vi "soundwave_generator_v01_only_player.vi"() -> ()   [LabVIEW 2019]
uses:
  <vilib>/sound2/lvsound2.llb/Sound Data Format.ctl
  <vilib>/sound2/lvsound2.llb/Sampling Mode.ctl
  <vilib>/Platform/TimedLoop/XDataNode/timing_clust.ctl
  <vilib>/Platform/TimedLoop/XDataNode/nitl_modes.ctl
  <vilib>/Platform/TimedLoop/XDataNode/wakeup.ctl
  <vilib>/sound2/lvsound2.llb/Sound Output Set Volume (Single).vi
  <vilib>/sound2/lvsound2.llb/Sound Output Write (DBL Single).vi
  <vilib>/platform/TimedLoop/XDataNode/XDataNode.xnode
  <vilib>/Platform/TimedLoop/XDataNode/XDNodeRunTimeDep.lvlib
panel:
  in  "frequency 2":dbl=440.0
  in  "volume 2":dbl(slide)=50.0 scale=0.0..100.0
  in  "play button 2":bool
  in  "play button 1":bool
  in  "frequency 1":dbl=440.0
  in  "volume 1":dbl(slide)=50.0 scale=0.0..100.0
  in  "stop":bool
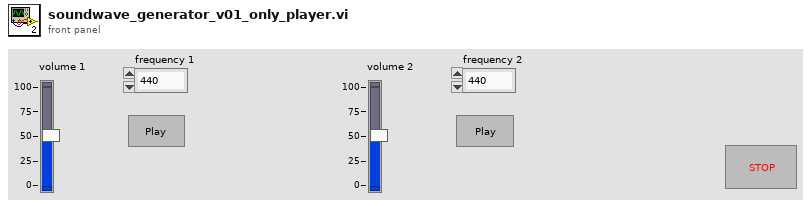
[diagram p1: front panel]
types:
  T1 = typedef "Sound Data Format.ctl" = cluster{"sample rate (S/s)":dbl, "number of channels":i32, "bits per sample":i32}
  T2 = typedef "XDNodeRunTimeDep.lvlib/timing_clust.ctl" = cluster{"Expected End [f-1]":u64, "Actual End [f-1]":u64, "Finished Late? [f-1]":bool, "Expected End [i-1]":u64, "Actual End [i-1]":u64, "Finished Late? [i-1]":bool, "Expected Start [i]":u64, "Actual Start [i]":u64, "Expected Start [f]":u64, "Actual Start [f]":u64, "Source Name":string, "Structure Name":string, "Period":i64, "Deadline":i64, "Offset":i64, "Start":i64, "Priority":i32, "Timeout":i32, "Mode":T3, "Wakeup Reason":T4, "Error":errorcluster, "Source Type":string, "Secondary Source Type":string, "Global End Time":u64, "Global Start Time":u64, "Frame Duration":u64, "Iteration Duration":u64, "Assigned CPU":i32, "I/O Scan Engine Mode":u32}
  T3 = typedef "XDNodeRunTimeDep.lvlib/nitl_modes.ctl" = enum32{"No Change", "Process missed periods, maintain original phase", "Discard missed periods, maintain original phase", "Process missed periods, ignore original phase", "Discard missed periods, ignore original phase"}
  T4 = typedef "XDNodeRunTimeDep.lvlib/wakeup.ctl" = enum32{"Normal", "Aborted", "Asynchronous wakeup", "Timing source error", "Timed loop error", "Timeout"}
  T5 = typedef "Sampling Mode.ctl" = i32
  T6 = typedef "Sound Output Task ID.ctl" = u32
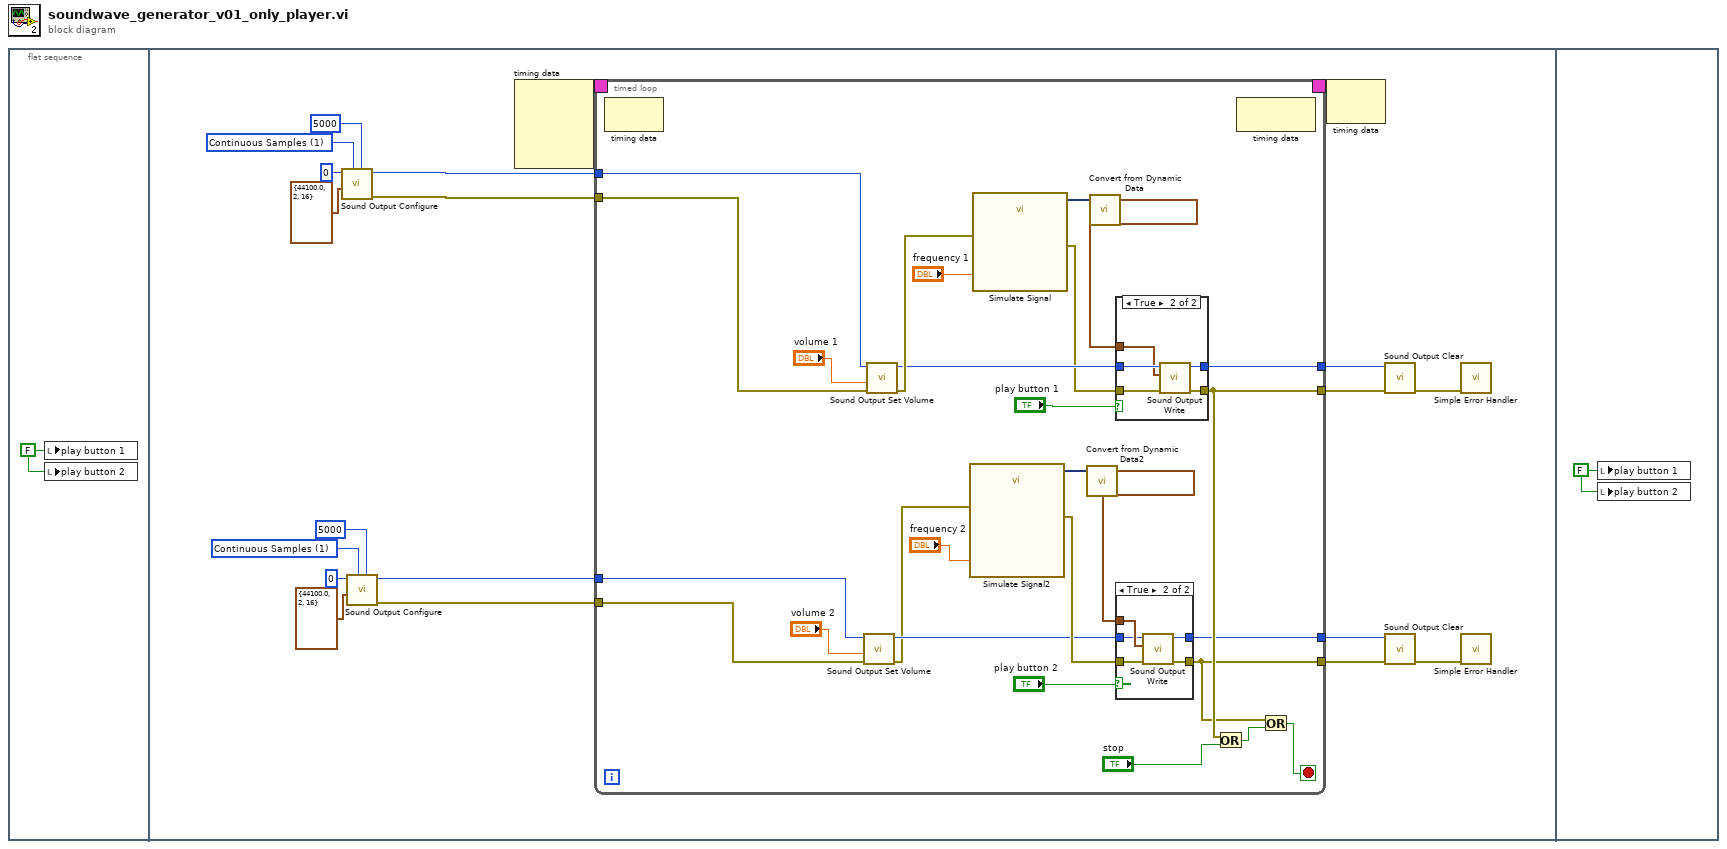
[diagram p0: block diagram]
diagram:
  n1 = flat-sequence {
    frame #0 {
      w1 = FALSE ("play button 1")
      n2 = local write "play button 1"(w1) -> ()
      n3 = local write "play button 2"(w1) -> ()
    }
    frame #1 {
      w4 = T5 1 items=["Finite Samples", "Continuous Samples"] ("sample mode")
      w9 = T5 1 items=["Finite Samples", "Continuous Samples"] ("sample mode")
      n4 = call <vilib>:"Sound Output Configure.vi"("number of samples/ch"=5000, "sample mode"=w9, "sound format"=T1 {"sample rate (S/s)"=44100.0, "number of channels"=2, "bits per sample"=16}, "device ID"=u32 0) -> ("error out"=w16:errorcluster, "task ID"=w15:T6)  [unwired: 6 in]
      n5 = call <vilib>:"Sound Output Configure.vi"("number of samples/ch"=5000, "sample mode"=w4, "sound format"=T1 {"sample rate (S/s)"=44100.0, "number of channels"=2, "bits per sample"=16}, "device ID"=u32 0) -> ("error out"=w12:errorcluster, "task ID"=w13:T6)  [unwired: 6 in]
      n6 = node-c288() -> (w21:T2)  [unwired: 4 in]
      n7 = timed-loop {
        tunnel: w16 -> [w44]
        tunnel: w15 -> [w46]
        tunnel: [w40] -> w19
        tunnel: [w37] -> w18
        tunnel: [w29] -> w10
        tunnel: [w28] -> w11
        tunnel: w13 -> [w27]
        tunnel: w12 -> [w26]
        timing: w21 -> [_]
        timing-out: [_] -> w20
        stop <- w22 stop-if-true
        n8 = node-c288() -> ()  [unwired: 1 in, 1 out]
        n9 = call-poly <vilib>:"Sound Output Set Volume.vi"("error in (no error)"=w26, "volume"="volume 2", "task ID"=w27) -> ("error out"=w31:errorcluster, "task ID out"=w33:T6)  [unwired: 7 in]
        n10 = call-poly <vilib>:"Sound Output Set Volume.vi"("error in (no error)"=w44, "volume"="volume 1", "task ID"=w46) -> ("error out"=w45:errorcluster, "task ID out"=w42:T6)  [unwired: 7 in]
        n11 = call "Simulate Signal2"("Frequency"="frequency 2", "error in (no error)"=w31) -> ("Sine"=w35:dynamicdata, "error out"=w34:errorcluster)  [unwired: 12 in]
        n12 = call "Simulate Signal"("Frequency"="frequency 1", "error in (no error)"=w45) -> ("Sine"=w39:dynamicdata, "error out"=w41:errorcluster)  [unwired: 12 in]
        n13 = call "Convert from Dynamic Data2"("Dynamic Data Type"=w35) -> ("Waveform"=w36:waveform(dbl))  [unwired: 3 in]
        n14 = call "Convert from Dynamic Data"("Dynamic Data Type"=w39) -> ("Waveform"=w38:waveform(dbl))  [unwired: 3 in]
        n15 = case shown="True" "play button 1" {
          tunnel: w42 -> [w59 w64]
          tunnel: w41 -> [w58 w63]
          tunnel: [w58 w62] -> w40
          tunnel: w38 -> [_ w61]
          tunnel: [w59 w60] -> w37
          frame False {
          }
          frame True {
            n16 = call-poly <vilib>:"Sound Output Write.vi"("error in (no error)"=w63, "data"=w61, "task ID"=w64) -> ("error out"=w62:errorcluster, "task ID out"=w60:T6)  [unwired: 7 in]
          }
        }
        n17 = case shown="True" "play button 2" {
          tunnel: w36 -> [_ w57]
          tunnel: w34 -> [w52 w56]
          tunnel: w33 -> [w51 w55]
          tunnel: [w52 w54] -> w29
          tunnel: [w51 w53] -> w28
          frame False {
          }
          frame True {
            n18 = call-poly <vilib>:"Sound Output Write.vi"("error in (no error)"=w56, "data"=w57, "task ID"=w55) -> ("error out"=w54:errorcluster, "task ID out"=w53:T6)  [unwired: 7 in]
          }
        }
        n19 = Or(x=w40, y="stop") -> (x .or. y?=w23:bool)
        n20 = node-c288() -> ()  [unwired: 1 in, 1 out]
        n21 = Or(x=w29, y=w23) -> (x .or. y?=w22:bool)
      }
      n22 = node-c288(w20) -> ()  [unwired: 1 out]
      n23 = call <vilib>:"Sound Output Clear.vi"("error in (no error)"=w19, "task ID"=w18) -> ("error out"=w17:errorcluster)  [unwired: 9 in]
      n24 = call <vilib>:"Sound Output Clear.vi"("error in (no error)"=w10, "task ID"=w11) -> ("error out"=w14:errorcluster)  [unwired: 9 in]
      n25 = call <vilib>:"Simple Error Handler.vi"("error in (no error)"=w17) -> ()  [unwired: 4 in, 5 out]
      n26 = call <vilib>:"Simple Error Handler.vi"("error in (no error)"=w14) -> ()  [unwired: 4 in, 5 out]
    }
    frame #2 {
      w67 = FALSE ("play button 1")
      n27 = local write "play button 1"(w67) -> ()
      n28 = local write "play button 2"(w67) -> ()
    }
  }
